vi "myfirst1.vi"() -> ()   [LabVIEW 2020]
panel:
  out "String 2":string
  in  "String":string
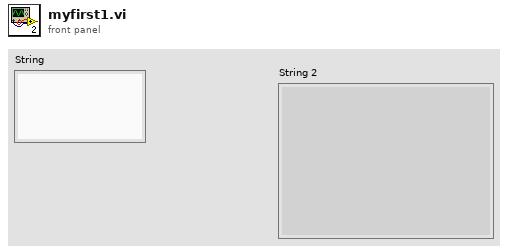
[diagram p1: front panel]
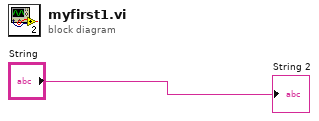
[diagram p0: block diagram]
diagram:
  "String 2" <- "String"
